vi "TestQueueTransport_ValueOK.vi"(8 "error in (no error)":errorcluster, 11 "TestCase in":refnum<class "TestTransport.lvclass">) -> (0 "error out":errorcluster, 3 "TestCase out":refnum<class "TestTransport.lvclass">)   [LabVIEW 2015, in "Transport.lvlib" / "TestTransport.lvclass"]
uses:
  TestTransport.lvclass
  QueueTransport/QueueTransport.lvclass
panel:
  out "element":T1
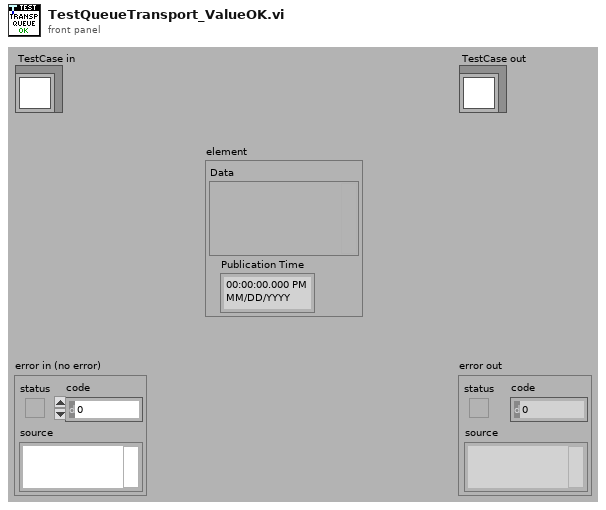
[diagram p1: front panel]
types:
  T1 = cluster{"Data":variant, "Publication Time":timestamp}
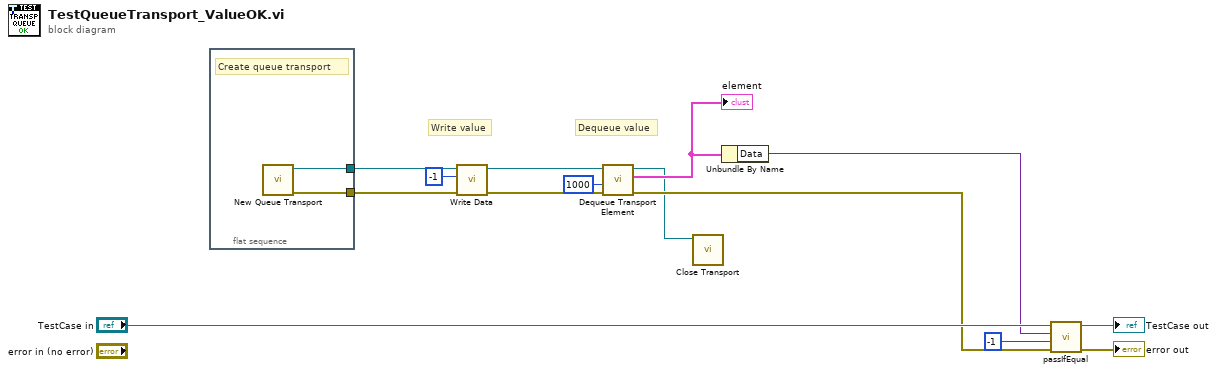
[diagram p0: block diagram]
diagram:
  # "Write value"
  # "Dequeue value"
  n1 = flat-sequence {
    tunnel: [w16] -> w9
    tunnel: [w15] -> w8
    frame #0 {
      # "Create queue transport"
      n2 = call "New Queue Transport.vi"() -> ("error out"=w15:errorcluster, "QueueTransport Out"=w16:refnum<class "QueueTransport.lvclass">)  [unwired: 10 in]
    }
  }
  n3 = call-dynamic "Write Data.vi"("error in (no error)"=w8, "Value"=-1, "QueueTransport In"=w9) -> ("error out"=w7:errorcluster, "QueueTransport Out"=w3:refnum<class "QueueTransport.lvclass">)  [unwired: 7 in]
  n4 = call "Dequeue Transport Element.vi"("error in (no error)"=w7, "Timeout In ms (-1)"=1000, "QueueTransport in"=w3) -> ("error out"=w6:errorcluster, "Element"=w5:T1, "QueueTransport out"=w1:refnum<class "QueueTransport.lvclass">)  [unwired: 5 in, 1 out]
  "element" <- w5
  n5 = call-dynamic "Close Transport.vi"("QueueTransport in"=w1) -> ()  [unwired: 10 in, 1 out]
  n6 = Unbundle By Name(w5) -> ("Data"=w4:variant)
  n7 = call-dynamic "passIfEqual.vi"("error in (no error)"=w6, "y"=-1, "x"=w4, "TestCase in"="TestCase in") -> ("error out"=→"error out":errorcluster, "TestCase out"=→"TestCase out":refnum<class "TestTransport.lvclass">)  [unwired: 6 in]
